vi "Initialization.vi"(8 "error in (no error)":errorcluster, 11 "Sensor in":refnum<class "Sensor.lvclass">) -> (0 "error out":errorcluster, 3 "Sensor Out":refnum<class "Sensor.lvclass">)   [LabVIEW 2018, in "Sensor.lvlib" / "Sensor.lvclass"]
uses:
  Sensor.lvclass
  Sensor.lvclass/Sensor.ctl
  PPLs/Configuration/Configuration.lvlibp/Configuration.lvclass
panel:
  in  "PPLs Folder Path":path
  in  "INI File Path":path
  in  "Device":string
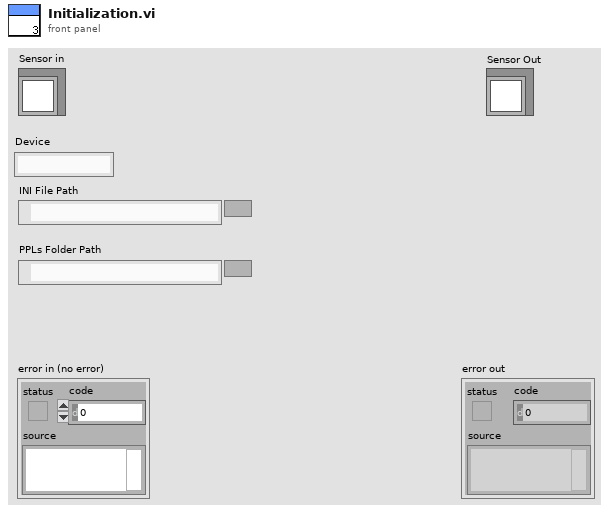
[diagram p1: front panel]
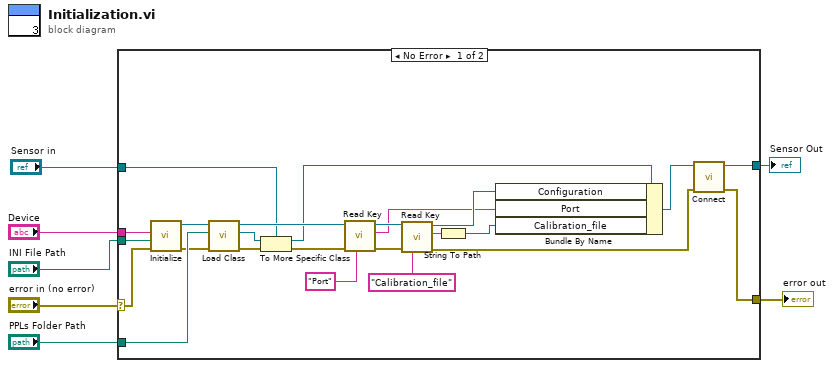
[diagram p0: block diagram]
diagram:
  n1 = case shown="No Error" "error in (no error)" {
    selector: "error in (no error)" -> [w24 w33]
    tunnel: [w8 w33] -> w6
    tunnel: [w16 w32] -> w1
    tunnel: "Sensor in" -> [w28 w32]
    tunnel: "Device" -> [w27 _]
    tunnel: "INI File Path" -> [w26 _]
    tunnel: "PPLs Folder Path" -> [w25 _]
    frame No Error {
      n2 = call "Initialize.vi"("error in"=w24, "INI File Path"=w26, "Device"=w27) -> ("error out"=w23:errorcluster, "Configuration out"=w31:refnum<class "Configuration.lvclass">)  [unwired: 7 in]
      n3 = call "Load Class.vi"("error in"=w23, "PPLs Folder Path"=w25, "Configuration in"=w31) -> ("error out"=w22:errorcluster, "Class out"=w29:refnum<class>, "Configuration out"=w30:refnum<class "Configuration.lvclass">)  [unwired: 6 in]
      n4 = To More Specific Class(target class=w28, reference=w29, error in=w22) -> (specific class reference=w18:refnum<class "Sensor.lvclass">, error out=w21:errorcluster)
      n5 = call "Read Key.vi"("Key:"="Port", "error in"=w21, "Configuration in"=w30) -> ("error out"=w20:errorcluster, "Value"=w12:string, "Configuration out"=w19:refnum<class "Configuration.lvclass">)  [unwired: 6 in]
      n6 = call "Read Key.vi"("Key:"="Calibration_file", "error in"=w20, "Configuration in"=w19) -> ("error out"=w9:errorcluster, "Value"=w11:string, "Configuration out"=w13:refnum<class "Configuration.lvclass">)  [unwired: 6 in]
      n7 = String To Path(string=w11) -> (path=w10:path)
      n8 = Bundle By Name(cluster=w18, "Configuration"=w13, "Port"=w12, "Calibration_file"=w10) -> (w17:refnum<class "Sensor.lvclass">)
      n9 = call-dynamic "Connect.vi"("error in (no error)"=w9, "Sensor in"=w17) -> ("error out"=w8:errorcluster, "Sensor out"=w16:refnum<class "Sensor.lvclass">)  [unwired: 7 in, 1 out]
    }
    frame Error {
    }
  }
  "error out" <- w6
  "Sensor Out" <- w1
